vi "Get Thermocouple Meas Volt.vi"(8 "error in (no error)":errorcluster, 11 "VISA resource name":refnum<visa-resource-name>) -> (0 "error out":errorcluster, 2 "Meas Value":dbl format="%^.3e", 3 "VISA resource name out":refnum<visa-resource-name>)   [LabVIEW 2011, in "Fluke 5XXX Series Multicalibrators.lvlib"]
doc: "This VI returns the last value of the thermocouple temperature measurement in volts. If the last measurement was an overload or open thermocouple condition, or there is no measurement, returns 0E+00.\n\nNote:\n\nThis VI is available only for instrument models 5500A and 5520A."
uses:
  Fluke 5XXX Series Multicalibrators.lvlib
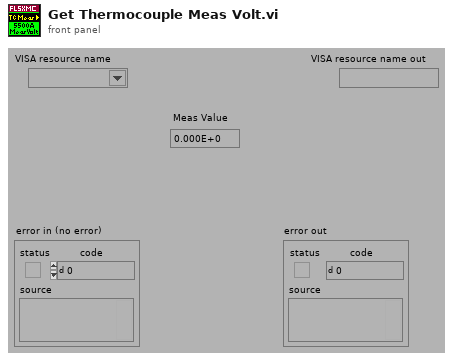
[diagram p1: front panel]
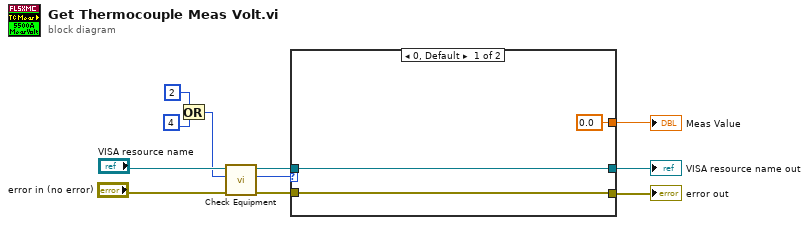
[diagram p0: block diagram]
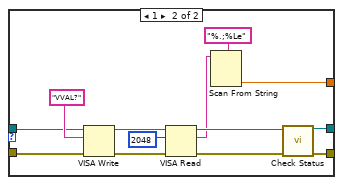
[diagram p2: hidden frame]
diagram:
  n1 = Or(x=2 ("Numeric"), y=4 ("Numeric")) -> (x .or. y?=w4:i32)
  n2 = call "Check Equipment.vi"("error in (no error)"="error in (no error)", "Bit Mask"=w4, "VISA resource name"="VISA resource name") -> ("error out"=w11:errorcluster, "Present?"=w9:u32, "VISA resource name out"=w10:refnum<visa-resource-name>)  [unwired: 6 in]
  n3 = case shown="0, Default" w9 {
    tunnel: [w14 w21] -> w2
    tunnel: [w13 w18] -> w1
    tunnel: w11 -> [w14 w23]
    tunnel: w10 -> [w13 w22]
    tunnel: [0.0 w15] -> w3
    frame 0, Default {
    }
    frame 1 {
      n4 = VISA Write(VISA resource name=w22, write buffer="VVAL?", error in (no error)=w23) -> (VISA resource name out=w26:refnum<visa-resource-name>, error out=w25:errorcluster)  [unwired: 1 out]
      n5 = VISA Read(VISA resource name=w26, byte count=u32 2048 ("byte count (0)"), error in (no error)=w25) -> (VISA resource name out=w19:refnum<visa-resource-name>, read buffer=w16:string, error out=w20:errorcluster)  [unwired: 1 out]
      n6 = Scan From String(format string="%.;%Le", input string=w16) -> (output 1=w15:dbl)  [unwired: 3 in, 3 out]
      n7 = call "Check Status.vi"("VISA resource name"=w19, "error in (no error)"=w20) -> ("VISA resource name out"=w18:refnum<visa-resource-name>, "error out"=w21:errorcluster)  [unwired: 12 in]
    }
  }
  "Meas Value" <- w3
  "VISA resource name out" <- w1
  "error out" <- w2
